vi "regGenUserEvent.vi"(8 "error in (no error)":errorcluster, 11 "tcpServerBase in":refnum<class "TcpServerBase.lvclass">) -> (0 "error out":errorcluster, 3 "tcpServerBase out":refnum<class "TcpServerBase.lvclass">)   [LabVIEW 2018, in "TcpServerBase.lvclass"]
doc: "Register the generic user event."
uses:
  TcpServerBase.lvclass
  TcpServerBase.lvclass/TcpServerBase.ctl
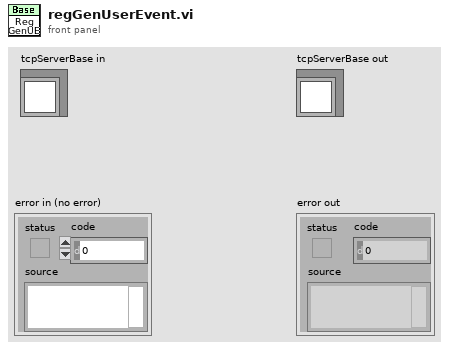
[diagram p1: front panel]
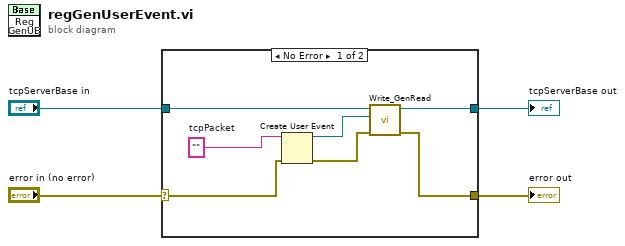
[diagram p0: block diagram]
diagram:
  n1 = case shown="No Error" "error in (no error)" {
    selector: "error in (no error)" -> [w6 w13]
    tunnel: [w5 w13] -> w3
    tunnel: [w10 w12] -> w1
    tunnel: "tcpServerBase in" -> [w11 w12]
    frame No Error {
      w7 = ""  # tcpPacket
      n2 = Create User Event(user event datatype=w7, error in=w6) -> (user event=w9:refnum<user-event>, error out=w8:errorcluster)
      n3 = call "Write_GenRead.vi"("error in (no error)"=w8, "GenRead"=w9, "TcpServerBase in"=w11) -> ("error out"=w5:errorcluster, "TcpServerBase out"=w10:refnum<class "TcpServerBase.lvclass">)  [unwired: 7 in]
    }
    frame Error {
    }
  }
  "error out" <- w3
  "tcpServerBase out" <- w1
